vi "Autonomous Independent.vi"() -> ()   [LabVIEW 2015]
doc: "This VI is called when autonomous begins, and will automatically be terminated when autonomous ends. You can carry out timed or sensor driven robot movement independently without needing to return to the caller."
uses:
  <vilib>/Rock Robotics/WPI/Utilities/WPI_GetSetVariantRefNum.vi
  <vilib>/Rock Robotics/Network Tables/NT Read String.vi
  <vilib>/Rock Robotics/Network Tables/NT Write Numeric Array.vi
  <vilib>/Rock Robotics/Network Tables/NT Write Number.vi
  <vilib>/addons/control/pid/pid.llb/PID (DBL).vi
  Robot Global Data.vi
  <vilib>/Rock Robotics/Network Tables/NT Read Number.vi
  <vilib>/addons/control/pid/NI_PID_pid.lvlib
  navX Library v2/navX Library v2.lvlib
panel:
  in  "Aiming Gains":T1={"proportional gain (Kc)"=1.0, "integral time (Ti, min)"=0.01, "derivative time (Td, min)"=0.0} {"derivative time (Td, min)" format="%.3f"; "integral time (Ti, min)" format="%.3f"; "proportional gain (Kc)" format="%.3f"}
  out "Yaw":dbl(graph)
  in  "Target Angle":dbl=30.0
  out "E1 Rate":dbl
  out "E2 Rate":dbl
  out "Yaw Display":dbl
  in  "Single Turn Gains":T1={"proportional gain (Kc)"=0.12, "integral time (Ti, min)"=0.0, "derivative time (Td, min)"=0.0} {"derivative time (Td, min)" format="%.3f"; "integral time (Ti, min)" format="%.3f"; "proportional gain (Kc)" format="%.3f"}
  in  "Yaw":T1={"proportional gain (Kc)"=0.2, "integral time (Ti, min)"=0.0, "derivative time (Td, min)"=0.0} {"derivative time (Td, min)" format="%.3f"; "integral time (Ti, min)" format="%.3f"; "proportional gain (Kc)" format="%.3f"}
  out "Right Motor Speed":dbl(graph)
  out "Left Motor Speed":dbl(graph)
  out "Right Motor":dbl(graph)
  out "Left Motor":dbl(graph)
  in  "Distance":dbl=120.0
  in  "Speed Gains":T1={"proportional gain (Kc)"=0.65, "integral time (Ti, min)"=0.001, "derivative time (Td, min)"=0.001} {"derivative time (Td, min)" format="%.3f"; "integral time (Ti, min)" format="%.3f"; "proportional gain (Kc)" format="%.3f"}
  out "E2 Dist":dbl
  out "E1 Dist":dbl
  # "Be sure to right-click and choose Data Operations>>Make Current Value default if you want to save the array values with the VI"
  # "Encoder Distance Traveled"
  # "Speed we are assigning the motors and Encoder Rate"
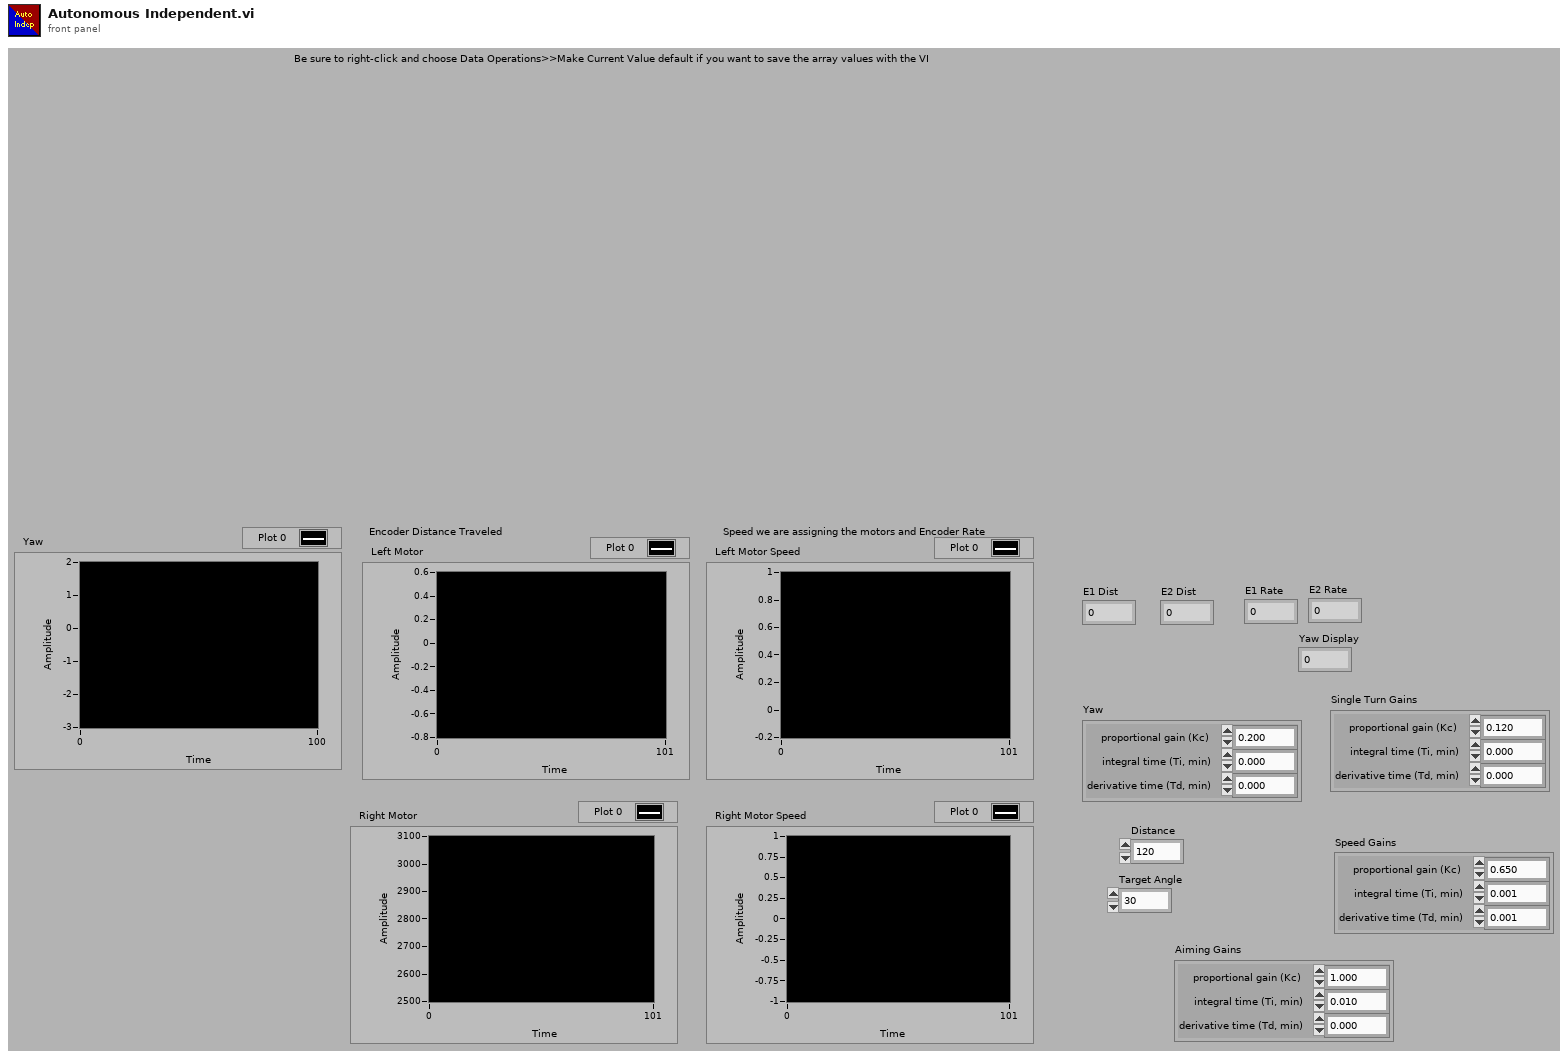
[diagram p1: front panel]
types:
  T1 = cluster{"proportional gain (Kc)":dbl, "integral time (Ti, min)":dbl, "derivative time (Td, min)":dbl}
  T2 = typedef "WPI_JoystickDevRef.ctl" = cluster{"Device":T3}
  T3 = typedef "WPI_JoystickDeviceEnum.ctl" = enum16{"USB 0", "USB 1", "USB 2", "USB 3", "USB 4", "USB 5"}
  T4 = typedef "navX Library v2.lvlib/Z900_navX_DeviceTypeDef.ctl" = cluster{"Interface":cluster{"Protocol":T5, "Update Rate (4Hz-60Hz)":u8, "navX Open TypeDef":variant}, "Notify Packet":refnum<notifier>, "Loop VI Refnum":refnum<vi>, "Ready to Close Occurrence Refnum":refnum<k4>}
  T5 = typedef "navX Library v2.lvlib/Z900_navX_ProtocolTypeDef.ctl" = enum16{"SERIAL", "I2C", "SPI"}
  T6 = typedef "WPI_EncoderDevRef.ctl" = cluster{"DevStatus":errorcluster, "EncoderIndex":T7, "CounterIndex":T8, "DistancePerCount":dbl, "Decoding Type":T9}
  T7 = typedef "FPGA_EncoderIdx.ctl" = enum8{"Enc 0", "Enc 1", "Enc 2", "Enc 3", "Enc 4", "Enc 5", "Enc 6", "Enc 7", "Invalid"}
  T8 = typedef "FPGA_CounterCtrSystemIndex.ctl" = enum8{"Ctr 0", "Ctr 1", "Ctr 2", "Ctr 3", "Ctr 4", "Ctr 5", "Ctr 6", "Ctr 7", "Invalid"}
  T9 = typedef "WPI_EncoderType.ctl" = enum16{"1x", "2x", "4x"}
  T10 = cluster{"Yaw":dbl, "Roll":dbl, "Pitch":dbl, "Heading":dbl, "Fused Heading":dbl}
  T11 = typedef "WPI_RobotDriveDevRef.ctl" = cluster{"DevStatus":errorcluster, "Motors[]":T12[], "Square Inputs":bool, "Max Output":dbl}
  T12 = typedef "WPI_MotorControlDeviceRef.ctl" = cluster{"DeviceStatus":errorcluster, "Type":T13, "PWM":cluster{"PWM Channel":T14, "DeadBand":T15}, "CAN":cluster{"Device Number":u8, "Control Mode":T16, "Semaphore":T17, "Max Vout":dbl, "TalonSRX Control Mode":T18}, "Invert":bool}
  T13 = typedef "WPI_MotorControlType.ctl" = enum16{"PWM", "CAN", "CANTalonSRX"}
  T14 = typedef "FPGA_DIOPWMChannel.ctl" = enum8{"PWM 0", "PWM 1", "PWM 2", "PWM 3", "PWM 4", "PWM 5", "PWM 6", "PWM 7", "PWM 8", "PWM 9", "PWM MXP 0", "PWM MXP 1", "PWM MXP 2", "PWM MXP 3", "PWM MXP 4", "PWM MXP 5", "PWM MXP 6", "PWM MXP 7", "PWM MXP 8", "PWM MXP 9", "Invalid"}
  T15 = typedef "WPI_PWMDeadband.ctl" = cluster{"Name":string, "maxPositivePwm":i32, "minPositivePwm":i32, "centerPwm":i32, "maxNegativePwm":i32, "minNegativePwm":i32, "angularRange":u16}
  T16 = typedef "WPI_CANJaguar_ControlMode.ctl" = enum8{"Percent VBus", "Current", "Speed", "Position", "Voltage"}
  T17 = typedef "Semaphore RefNum" = refnum<k1>
  T18 = typedef "WPI_CANTalonSRX_APIControlMode.ctl" = enum8{"Percent VBus", "Speed", "Position", "Slave", "Unchanged / Invalid", "Voltage Compensation", "Current", "Motion Profile"}
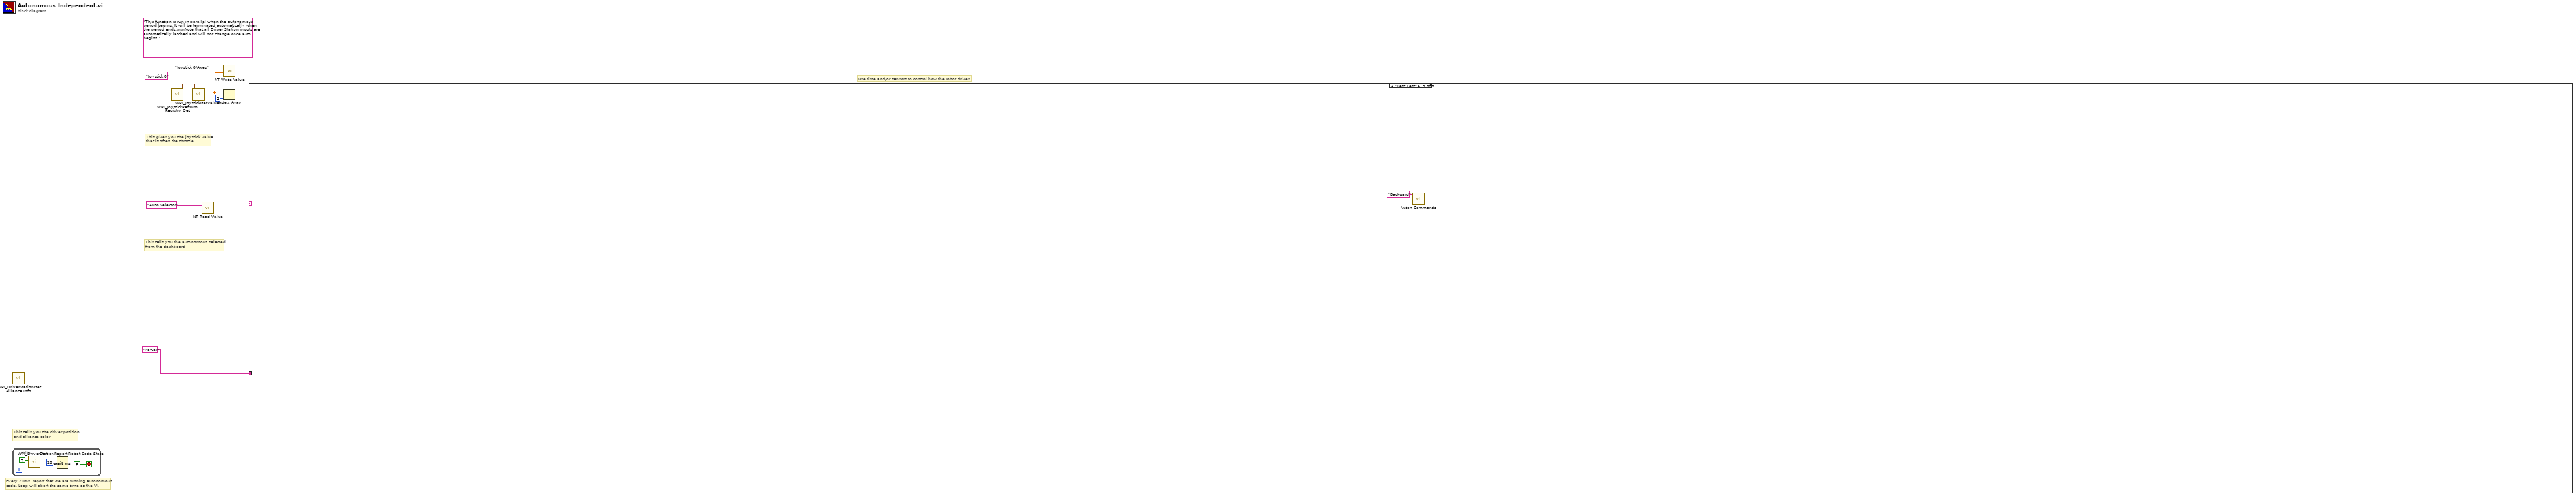
[diagram p0: block diagram]
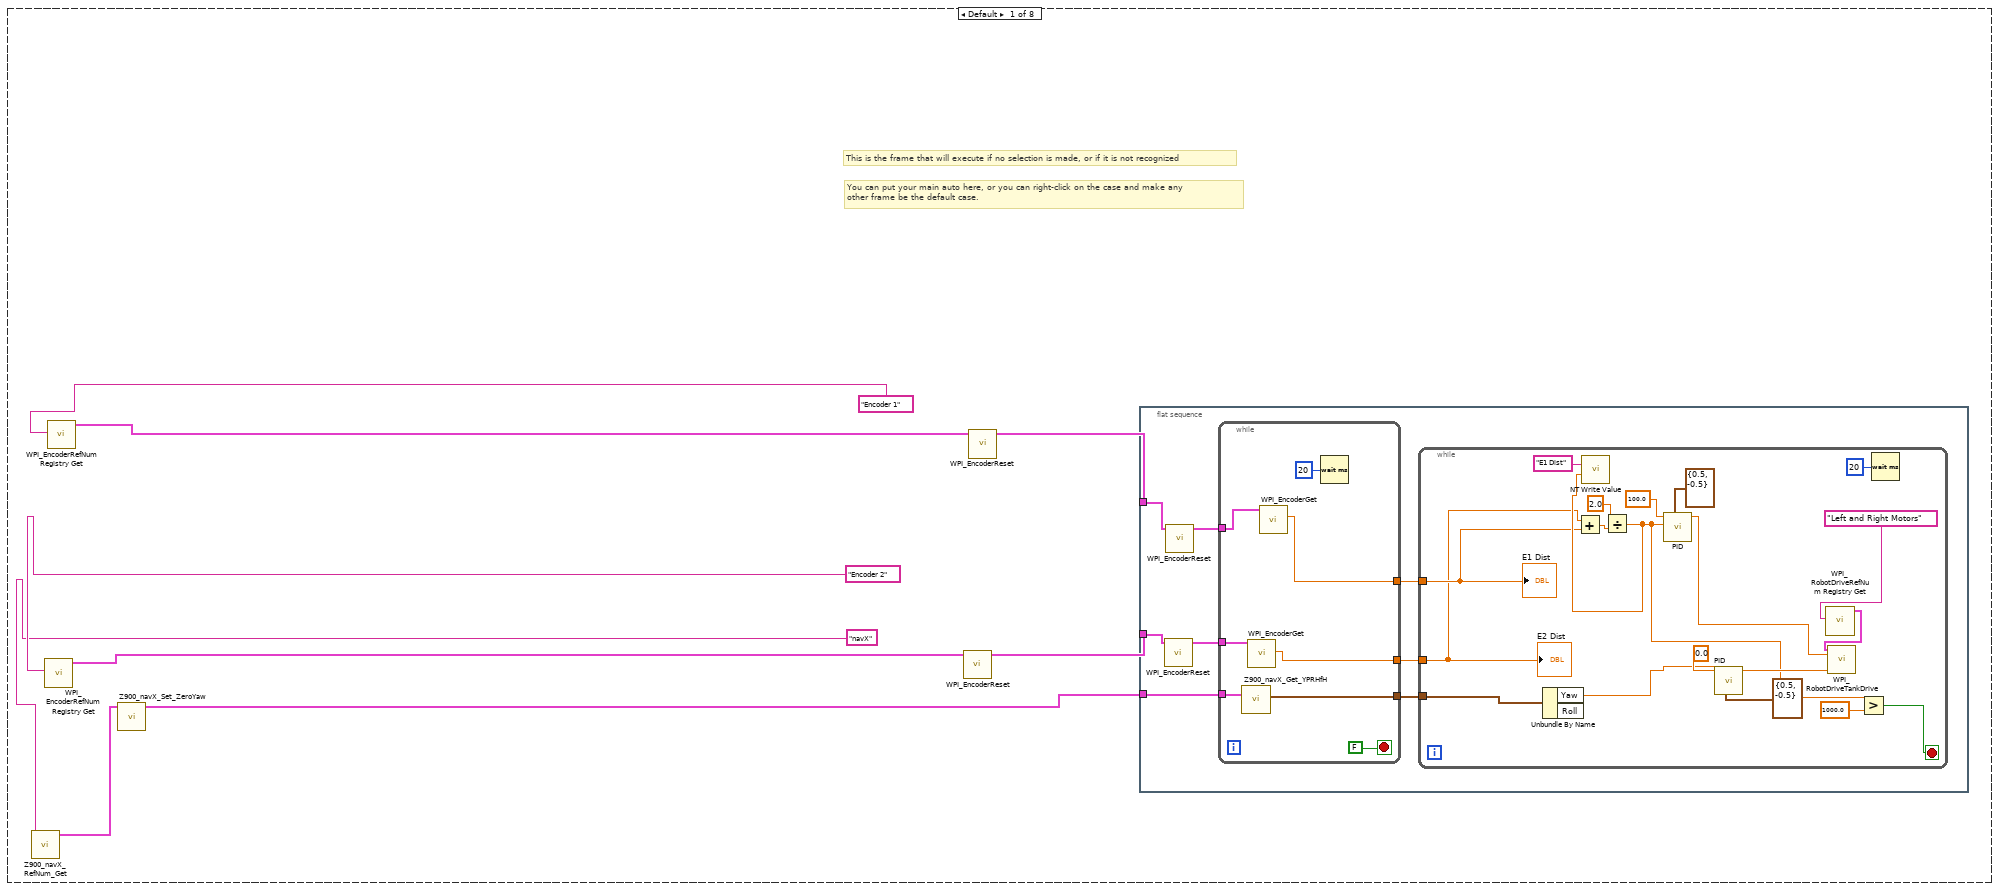
[diagram p2: hidden frame]
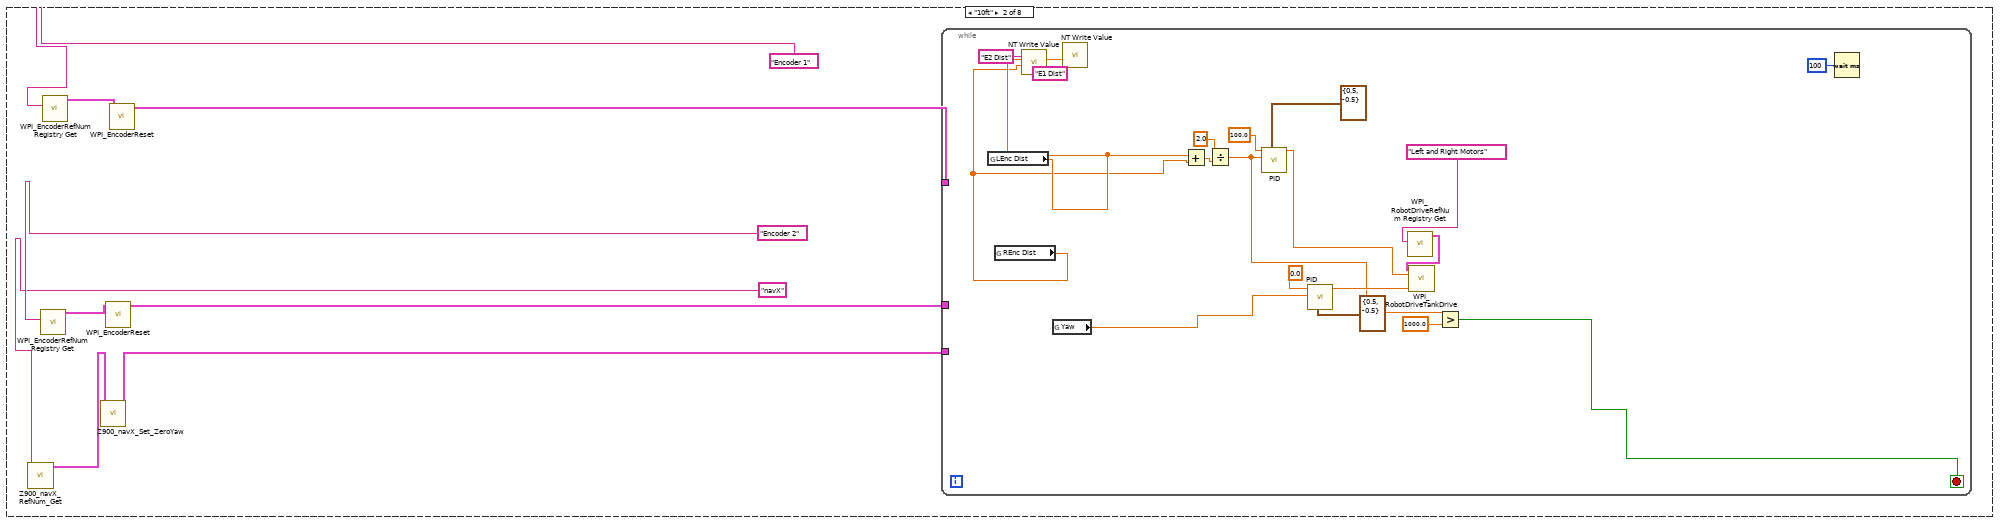
[diagram p3: hidden frame]
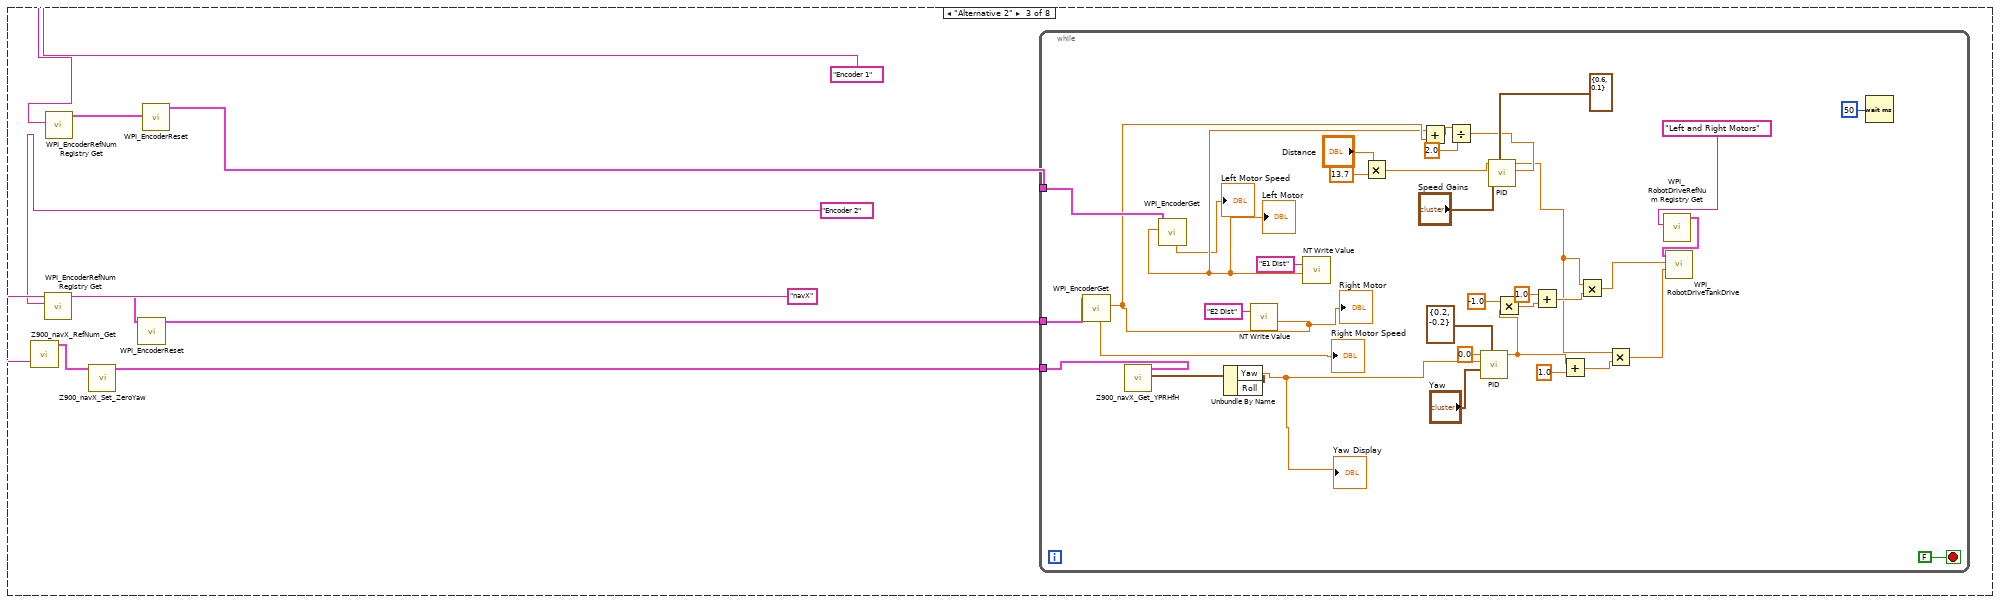
[diagram p4: hidden frame]
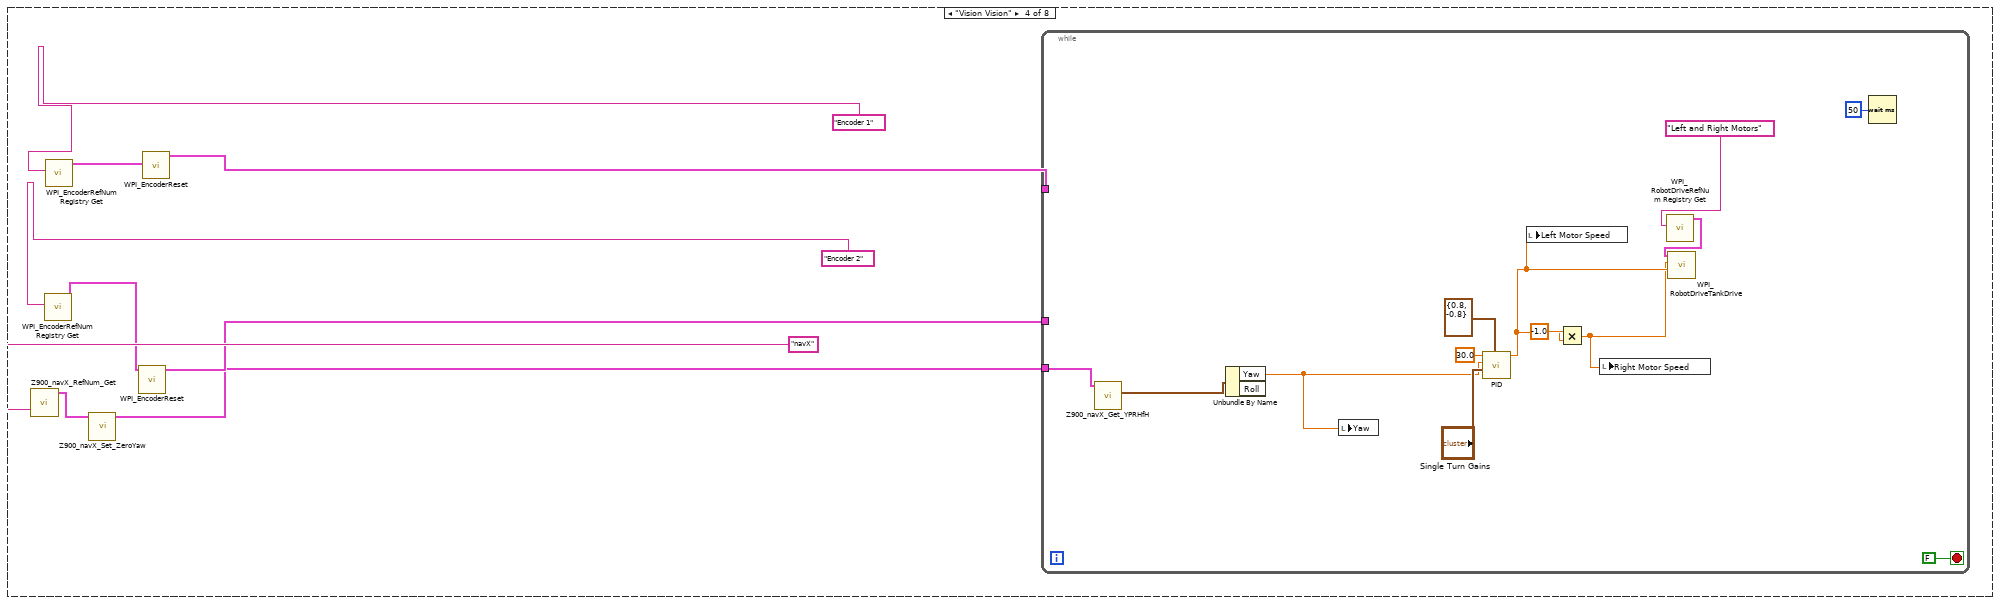
[diagram p5: hidden frame]
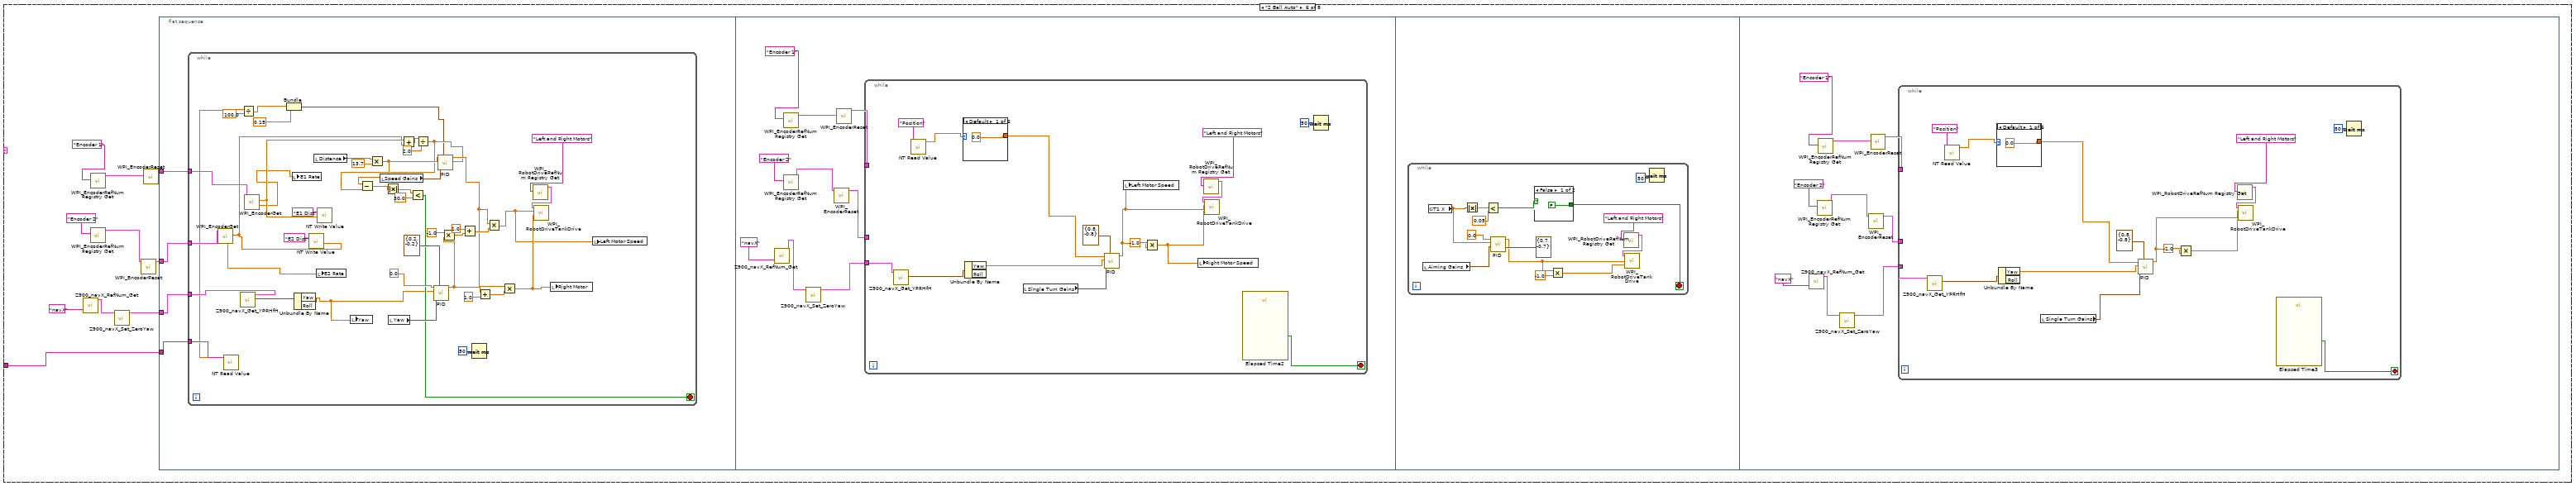
[diagram p6: hidden frame]
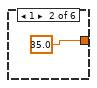
[diagram p7: hidden frame]
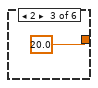
[diagram p8: hidden frame]
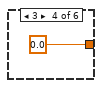
[diagram p9: hidden frame]
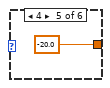
[diagram p10: hidden frame]
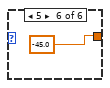
[diagram p11: hidden frame]
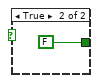
[diagram p12: hidden frame]
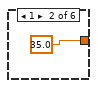
[diagram p13: hidden frame]
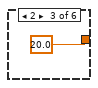
[diagram p14: hidden frame]
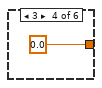
[diagram p15: hidden frame]
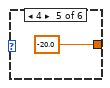
[diagram p16: hidden frame]
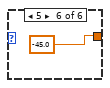
[diagram p17: hidden frame]
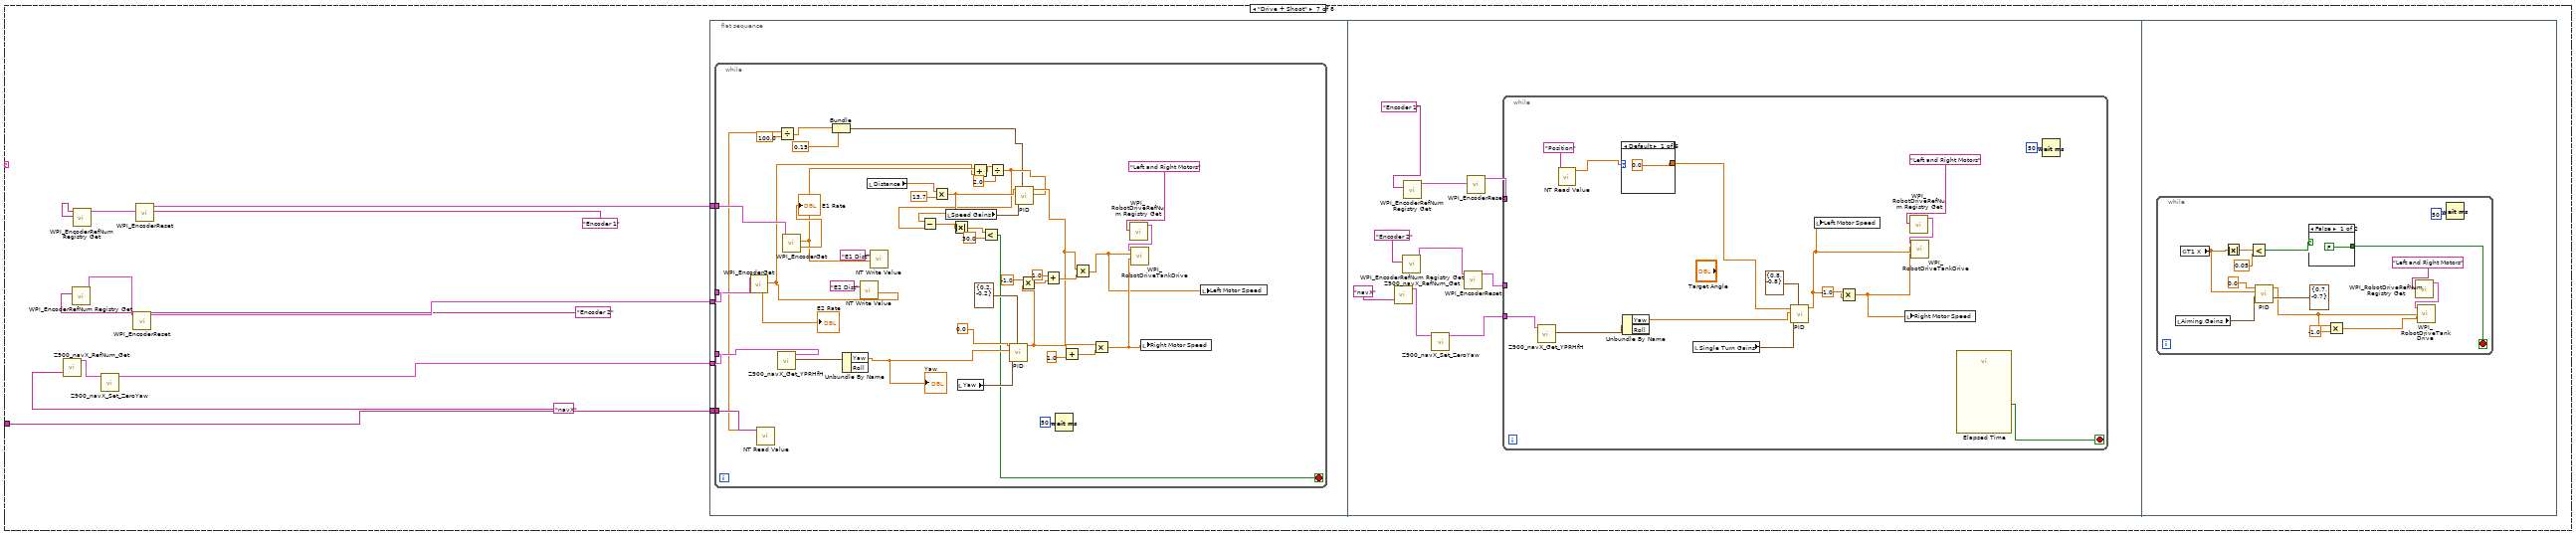
[diagram p18: hidden frame]
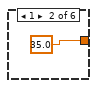
[diagram p19: hidden frame]
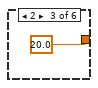
[diagram p20: hidden frame]
diagram:
  (unwired) "This function is run in parallel when the autonomous period begins. It will be terminated automatically when the period ends.\n\nNote that all Driver Station inputs are automatically latched and will not change once auto begins."
  # "This tells you the autonomous selected\nfrom the dashboard"
  # "Every 20ms, report that we are running autonomous\ncode. Loop will abort the same time as the VI."
  # "This gives you the joystick value\nthat is often the throttle"
  # "Use time and/or sensors to control how the robot drives."
  # "This tells you the driver position\nand alliance color"
  n1 = while {
    stop <- FALSE stop-if-true
    n2 = call <vilib>:"WPI_DriverStationReport Robot Code State.vi"("Autonomous"=TRUE) -> ()  [unwired: 10 in, 1 out]
    n3 = Wait (ms)(milliseconds to wait=u32 20) -> ()  [unwired: 1 out]
  }
  n4 = call <vilib>:"WPI_DriverStationGet Alliance Info.vi"() -> ()  [unwired: 12 out]
  n5 = call <vilib>:"WPI_JoystickRefNum Registry Get.vi"("refnum name"="Joystick 0") -> ("JoystickDevRef"=w7:T2)  [unwired: 1 in, 9 out]
  n6 = call <vilib>:"WPI_JoystickGetValues.vi"("JoystickDevRef"=w7) -> ("Axes"=w3:dbl[])  [unwired: 6 in, 4 out]
  n7 = call-poly <vilib>:"NT Read Value.vi"("Name"="Auto Selector") -> ("String"=w4:string)  [unwired: 9 in, 1 out]
  n8 = call-poly <vilib>:"NT Write Value.vi"("Numeric Array"=w3, "Name"="Joystick 0/Axes") -> ()  [unwired: 9 in, 1 out]
  n9 = Index Array(array=w3, index=2) -> ()  [unwired: 1 out]
  n10 = case shown="\"Test Test\"" w4 {
    tunnel: "Power" ("Name") -> [_ _ _ _ _ w152 w286 _]
    frame Default {
      # "You can put your main auto here, or you can right-click on the case and make any\nother frame be the default case."
      # "This is the frame that will execute if no selection is made, or if it is not recognized"
      n11 = call "Z900_navX_RefNum_Get.vi"("refnum name"="navX") -> ("navX Device"=w14:T4)  [unwired: 9 in, 1 out]
      n12 = call <vilib>:"WPI_EncoderRefNum Registry Get.vi"("refnum name"="Encoder 2") -> ("EncoderDevRef"=w16:T6)  [unwired: 9 in, 1 out]
      n13 = call <vilib>:"WPI_EncoderRefNum Registry Get.vi"("refnum name"="Encoder 1") -> ("EncoderDevRef"=w18:T6)  [unwired: 9 in, 1 out]
      n14 = call "Z900_navX_Set_ZeroYaw.vi"("navX Device"=w14) -> ("navX Device"=w13:T4)  [unwired: 9 in, 1 out]
      n15 = call <vilib>:"WPI_EncoderReset.vi"("EncoderDevRef"=w16) -> ("EncoderDevRef"=w15:T6)  [unwired: 9 in, 1 out]
      n16 = call <vilib>:"WPI_EncoderReset.vi"("EncoderDevRef"=w18) -> ("EncoderDevRef"=w17:T6)  [unwired: 9 in, 1 out]
      n17 = flat-sequence {
        tunnel: w17 -> [w28]
        tunnel: w15 -> [w27]
        tunnel: w13 -> [w26]
        frame #0 {
          n18 = call <vilib>:"WPI_EncoderReset.vi"("EncoderDevRef"=w27) -> ("EncoderDevRef"=w25:T6)  [unwired: 9 in, 1 out]
          n19 = call <vilib>:"WPI_EncoderReset.vi"("EncoderDevRef"=w28) -> ("EncoderDevRef"=w24:T6)  [unwired: 9 in, 1 out]
          n20 = while {
            tunnel: w26 -> [w33]
            tunnel: w25 -> [w34]
            tunnel: w24 -> [w35]
            tunnel: [w32] -> w23
            tunnel: [w31] -> w22
            tunnel: [w30] -> w21
            stop <- FALSE stop-if-true
            n21 = call "Z900_navX_Get_YPRHfH.vi"("navX Device"=w33) -> ("YRPHfH"=w32:T10)  [unwired: 7 in, 3 out]
            n22 = call <vilib>:"WPI_EncoderGet.vi"("EncoderDevRef"=w34) -> ("Distance"=w31:dbl)  [unwired: 5 in, 5 out]
            n23 = call <vilib>:"WPI_EncoderGet.vi"("EncoderDevRef"=w35) -> ("Distance"=w30:dbl)  [unwired: 5 in, 5 out]
            n24 = Wait (ms)(milliseconds to wait=u32 20) -> ()  [unwired: 1 out]
          }
          n25 = while {
            tunnel: w23 -> [w40]
            tunnel: w22 -> [w38]
            tunnel: w21 -> [w39]
            stop <- w44 stop-if-true
            n26 = Unbundle By Name(w40) -> ("Yaw"=w41:dbl)  [unwired: 1 out]
            n27 = Add(x=w38, y=w39) -> (x+y=w55:dbl)
            n28 = Divide(x=2.0, y=w55) -> (x/y=w43:dbl)
            n29 = call-poly <vilib>:"NT Write Value.vi"("Numeric"=w43, "Name"="E1 Dist") -> ()  [unwired: 9 in, 1 out]
            n30 = call-poly <vilib>:"PID.vi"("output range"=cluster{"output high":dbl, "output low":dbl} {"output high"=0.5, "output low"=-0.5}, "process variable"=w43, "setpoint"=100.0) -> ("output"=w48:dbl)  [unwired: 7 in, 1 out]
            n31 = call-poly <vilib>:"PID.vi"("output range"=cluster{"output high":dbl, "output low":dbl} {"output high"=0.5, "output low"=-0.5}, "process variable"=w41, "setpoint"=0.0) -> ("output"=w47:dbl)  [unwired: 7 in, 1 out]
            n32 = call <vilib>:"WPI_RobotDriveRefNum Registry Get.vi"("refnum name"="Left and Right Motors") -> ("RobotDriveDevRef"=w50:T11)  [unwired: 9 in, 1 out]
            n33 = call <vilib>:"WPI_RobotDriveTankDrive.vi"("Right axis value"=w47, "Left axis value"=w48, "RobotDriveDevRef"=w50) -> ()  [unwired: 6 in, 3 out]
            n34 = Greater?(x=w43, y=1000.0) -> (0:w44:bool)
            n35 = Wait (ms)(milliseconds to wait=u32 20) -> ()  [unwired: 1 out]
            "E2 Dist" <- w38
            "E1 Dist" <- w39
          }
        }
      }
    }
    frame "10ft" {
      n36 = call "Z900_navX_RefNum_Get.vi"("refnum name"="navX") -> ("navX Device"=w58:T4)  [unwired: 9 in, 1 out]
      n37 = call <vilib>:"WPI_EncoderRefNum Registry Get.vi"("refnum name"="Encoder 2") -> ("EncoderDevRef"=w60:T6)  [unwired: 9 in, 1 out]
      n38 = call <vilib>:"WPI_EncoderRefNum Registry Get.vi"("refnum name"="Encoder 1") -> ("EncoderDevRef"=w62:T6)  [unwired: 9 in, 1 out]
      n39 = call "Z900_navX_Set_ZeroYaw.vi"("navX Device"=w58) -> ("navX Device"=w57:T4)  [unwired: 9 in, 1 out]
      n40 = call <vilib>:"WPI_EncoderReset.vi"("EncoderDevRef"=w60) -> ("EncoderDevRef"=w59:T6)  [unwired: 9 in, 1 out]
      n41 = call <vilib>:"WPI_EncoderReset.vi"("EncoderDevRef"=w62) -> ("EncoderDevRef"=w61:T6)  [unwired: 9 in, 1 out]
      n42 = while {
        tunnel: w61 -> [_]
        tunnel: w59 -> [_]
        tunnel: w57 -> [_]
        stop <- w65 stop-if-true
        n43 = global read "Robot Global Data.vi" "LEnc Dist"() -> (w68:dbl)
        n44 = global read "Robot Global Data.vi" "REnc Dist"() -> (w67:dbl)
        n45 = call-poly <vilib>:"NT Write Value.vi"("Numeric"=w67, "Name"="E2 Dist") -> ()  [unwired: 9 in, 1 out]
        n46 = global read "Robot Global Data.vi" "Yaw"() -> (w66:dbl)
        n47 = call-poly <vilib>:"NT Write Value.vi"("Numeric"=w68, "Name"="E1 Dist") -> ()  [unwired: 9 in, 1 out]
        n48 = Add(x=w68, y=w67) -> (x+y=w82:dbl)
        n49 = Divide(x=2.0, y=w82) -> (x/y=w72:dbl)
        n50 = call-poly <vilib>:"PID.vi"("output range"=cluster{"output high":dbl, "output low":dbl} {"output high"=0.5, "output low"=-0.5}, "process variable"=w72, "setpoint"=100.0) -> ("output"=w76:dbl)  [unwired: 7 in, 1 out]
        n51 = call-poly <vilib>:"PID.vi"("output range"=cluster{"output high":dbl, "output low":dbl} {"output high"=0.5, "output low"=-0.5}, "process variable"=w66, "setpoint"=0.0) -> ("output"=w75:dbl)  [unwired: 7 in, 1 out]
        n52 = call <vilib>:"WPI_RobotDriveRefNum Registry Get.vi"("refnum name"="Left and Right Motors") -> ("RobotDriveDevRef"=w78:T11)  [unwired: 9 in, 1 out]
        n53 = call <vilib>:"WPI_RobotDriveTankDrive.vi"("Right axis value"=w75, "Left axis value"=w76, "RobotDriveDevRef"=w78) -> ()  [unwired: 6 in, 3 out]
        n54 = Greater?(x=w72, y=1000.0) -> (0:w65:bool)
        n55 = Wait (ms)(milliseconds to wait=u32 100) -> ()  [unwired: 1 out]
      }
    }
    frame "Alternative 2" {
      n56 = call "Z900_navX_RefNum_Get.vi"("refnum name"="navX") -> ("navX Device"=w85:T4)  [unwired: 9 in, 1 out]
      n57 = call <vilib>:"WPI_EncoderRefNum Registry Get.vi"("refnum name"="Encoder 2") -> ("EncoderDevRef"=w87:T6)  [unwired: 9 in, 1 out]
      n58 = call <vilib>:"WPI_EncoderRefNum Registry Get.vi"("refnum name"="Encoder 1") -> ("EncoderDevRef"=w89:T6)  [unwired: 9 in, 1 out]
      n59 = call "Z900_navX_Set_ZeroYaw.vi"("navX Device"=w85) -> ("navX Device"=w84:T4)  [unwired: 9 in, 1 out]
      n60 = call <vilib>:"WPI_EncoderReset.vi"("EncoderDevRef"=w87) -> ("EncoderDevRef"=w86:T6)  [unwired: 9 in, 1 out]
      n61 = call <vilib>:"WPI_EncoderReset.vi"("EncoderDevRef"=w89) -> ("EncoderDevRef"=w88:T6)  [unwired: 9 in, 1 out]
      n62 = while {
        tunnel: w88 -> [w121]
        tunnel: w86 -> [w120]
        tunnel: w84 -> [w119]
        stop <- FALSE stop-if-true
        n63 = call <vilib>:"WPI_EncoderGet.vi"("EncoderDevRef"=w120) -> ("Distance"=w110:dbl, "Rate"=→"Right Motor Speed":dbl)  [unwired: 5 in, 4 out]
        "Right Motor" <- w110
        n64 = call "Z900_navX_Get_YPRHfH.vi"("navX Device"=w119) -> ("YRPHfH"=w122:T10)  [unwired: 7 in, 3 out]
        n65 = call <vilib>:"WPI_EncoderGet.vi"("EncoderDevRef"=w121) -> ("Distance"=w109:dbl, "Rate"=→"Left Motor Speed":dbl)  [unwired: 5 in, 4 out]
        "Left Motor" <- w109
        n66 = Unbundle By Name(w122) -> ("Yaw"=w95:dbl)  [unwired: 1 out]
        "Yaw Display" <- w95
        n67 = call-poly <vilib>:"NT Write Value.vi"("Numeric"=w110, "Name"="E2 Dist") -> ()  [unwired: 9 in, 1 out]
        n68 = call-poly <vilib>:"NT Write Value.vi"("Numeric"=w109, "Name"="E1 Dist") -> ()  [unwired: 9 in, 1 out]
        n69 = Multiply(x="Distance", y=13.7) -> (x*y=w111:dbl)
        n70 = Add(x=w109, y=w110) -> (x+y=w116:dbl)
        n71 = Divide(x=w116, y=2.0) -> (x/y=w114:dbl)
        n72 = call-poly <vilib>:"PID.vi"("output range"=cluster{"output high":dbl, "output low":dbl} {"output high"=0.2, "output low"=-0.2}, "PID gains"="Yaw", "process variable"=w95, "setpoint"=0.0) -> ("output"=w99:dbl)  [unwired: 6 in, 1 out]
        n73 = call-poly <vilib>:"PID.vi"("output range"=cluster{"output high":dbl, "output low":dbl} {"output high"=0.6, "output low"=0.1}, "PID gains"="Speed Gains", "process variable"=w114, "setpoint"=w111) -> ("output"=w96:dbl)  [unwired: 6 in, 1 out]
        n74 = Multiply(x=-1.0, y=w99) -> (x*y=w100:dbl)
        n75 = Add(x=1.0, y=w100) -> (x+y=w101:dbl)
        n76 = Add(x=w99, y=1.0) -> (x+y=w102:dbl)
        n77 = Multiply(x=w96, y=w101) -> (x*y=w93:dbl)
        n78 = Multiply(x=w96, y=w102) -> (x*y=w94:dbl)
        n79 = call <vilib>:"WPI_RobotDriveRefNum Registry Get.vi"("refnum name"="Left and Right Motors") -> ("RobotDriveDevRef"=w124:T11)  [unwired: 9 in, 1 out]
        n80 = call <vilib>:"WPI_RobotDriveTankDrive.vi"("Right axis value"=w94, "Left axis value"=w93, "RobotDriveDevRef"=w124) -> ()  [unwired: 6 in, 3 out]
        n81 = Wait (ms)(milliseconds to wait=u32 50) -> ()  [unwired: 1 out]
      }
    }
    frame "Vision Vision" {
      n82 = call "Z900_navX_RefNum_Get.vi"("refnum name"="navX") -> ("navX Device"=w130:T4)  [unwired: 9 in, 1 out]
      n83 = call <vilib>:"WPI_EncoderRefNum Registry Get.vi"("refnum name"="Encoder 2") -> ("EncoderDevRef"=w132:T6)  [unwired: 9 in, 1 out]
      n84 = call <vilib>:"WPI_EncoderRefNum Registry Get.vi"("refnum name"="Encoder 1") -> ("EncoderDevRef"=w134:T6)  [unwired: 9 in, 1 out]
      n85 = call "Z900_navX_Set_ZeroYaw.vi"("navX Device"=w130) -> ("navX Device"=w129:T4)  [unwired: 9 in, 1 out]
      n86 = call <vilib>:"WPI_EncoderReset.vi"("EncoderDevRef"=w132) -> ("EncoderDevRef"=w131:T6)  [unwired: 9 in, 1 out]
      n87 = call <vilib>:"WPI_EncoderReset.vi"("EncoderDevRef"=w134) -> ("EncoderDevRef"=w133:T6)  [unwired: 9 in, 1 out]
      n88 = while {
        tunnel: w133 -> [_]
        tunnel: w131 -> [_]
        tunnel: w129 -> [w144]
        stop <- FALSE stop-if-true
        n89 = call "Z900_navX_Get_YPRHfH.vi"("navX Device"=w144) -> ("YRPHfH"=w143:T10)  [unwired: 7 in, 3 out]
        n90 = Unbundle By Name(w143) -> ("Yaw"=w138:dbl)  [unwired: 1 out]
        n91 = local write "Yaw"(w138) -> ()
        n92 = call-poly <vilib>:"PID.vi"("output range"=cluster{"output high":dbl, "output low":dbl} {"output high"=0.8, "output low"=-0.8}, "PID gains"="Single Turn Gains", "process variable"=w138, "setpoint"=30.0) -> ("output"=w140:dbl)  [unwired: 6 in, 1 out]
        n93 = local write "Left Motor Speed"(w140) -> ()
        n94 = Multiply(x=-1.0, y=w140) -> (x*y=w139:dbl)
        n95 = local write "Right Motor Speed"(w139) -> ()
        n96 = call <vilib>:"WPI_RobotDriveRefNum Registry Get.vi"("refnum name"="Left and Right Motors") -> ("RobotDriveDevRef"=w149:T11)  [unwired: 9 in, 1 out]
        n97 = call <vilib>:"WPI_RobotDriveTankDrive.vi"("Right axis value"=w140, "Left axis value"=w139, "RobotDriveDevRef"=w149) -> ()  [unwired: 6 in, 3 out]
        n98 = Wait (ms)(milliseconds to wait=u32 50) -> ()  [unwired: 1 out]
      }
    }
    frame "Test Test" {
      n99 = call "Auton Commands.vi"("Task"="Backward") -> ()  [unwired: 10 in]
    }
    frame "2 Ball Auto" {
      n100 = call "Z900_navX_RefNum_Get.vi"("refnum name"="navX") -> ("navX Device"=w160:T4)  [unwired: 9 in, 1 out]
      n101 = call <vilib>:"WPI_EncoderRefNum Registry Get.vi"("refnum name"="Encoder 2") -> ("EncoderDevRef"=w158:T6)  [unwired: 9 in, 1 out]
      n102 = call <vilib>:"WPI_EncoderRefNum Registry Get.vi"("refnum name"="Encoder 1") -> ("EncoderDevRef"=w156:T6)  [unwired: 9 in, 1 out]
      n103 = call "Z900_navX_Set_ZeroYaw.vi"("navX Device"=w160) -> ("navX Device"=w161:T4)  [unwired: 9 in, 1 out]
      n104 = call <vilib>:"WPI_EncoderReset.vi"("EncoderDevRef"=w158) -> ("EncoderDevRef"=w159:T6)  [unwired: 9 in, 1 out]
      n105 = call <vilib>:"WPI_EncoderReset.vi"("EncoderDevRef"=w156) -> ("EncoderDevRef"=w157:T6)  [unwired: 9 in, 1 out]
      n106 = flat-sequence {
        tunnel: w161 -> [w165]
        tunnel: w159 -> [w164]
        tunnel: w157 -> [w163]
        tunnel: w152 -> [w162]
        frame #0 {
          n107 = while {
            tunnel: w163 -> [w203]
            tunnel: w164 -> [w202]
            tunnel: w165 -> [w201]
            tunnel: w162 -> [w175]
            stop <- w176 stop-if-true
            n108 = call <vilib>:"WPI_EncoderGet.vi"("EncoderDevRef"=w202) -> ("Distance"=w182:dbl, "Rate"=w167:dbl)  [unwired: 5 in, 4 out]
            n109 = call-poly <vilib>:"NT Read Value.vi"("Name"=w175) -> ("Numeric"=w174:dbl)  [unwired: 9 in, 1 out]
            n110 = call "Z900_navX_Get_YPRHfH.vi"("navX Device"=w201) -> ("YRPHfH"=w204:T10)  [unwired: 7 in, 3 out]
            n111 = Divide(x=w174, y=100.0) -> (x/y=w172:dbl)
            n112 = call <vilib>:"WPI_EncoderGet.vi"("EncoderDevRef"=w203) -> ("Distance"=w183:dbl, "Rate"=w166:dbl)  [unwired: 5 in, 4 out]
            n113 = Bundle(w172, "output low"=0.15) -> (w170:cluster{dbl, "output low":dbl})  [unwired: 1 in]
            n114 = local write "E1 Rate"(w166) -> ()
            n115 = Unbundle By Name(w204) -> ("Yaw"=w168:dbl)  [unwired: 1 out]
            n116 = call-poly <vilib>:"NT Write Value.vi"("Numeric"=w182, "Name"="E2 Dist") -> ()  [unwired: 9 in, 1 out]
            n117 = local read "Distance"() -> (w169:dbl)
            n118 = local write "E2 Rate"(w167) -> ()
            n119 = call-poly <vilib>:"NT Write Value.vi"("Numeric"=w183, "Name"="E1 Dist") -> ()  [unwired: 9 in, 1 out]
            n120 = local write "Yaw"(w168) -> ()
            n121 = Multiply(x=w169, y=13.7) -> (x*y=w181:dbl)
            n122 = local read "Speed Gains"() -> (w185:T1)
            n123 = local read "Yaw"() -> (w188:T1)
            n124 = Add(x=w183, y=w182) -> (x+y=w200:dbl)
            n125 = Divide(x=w200, y=2.0) -> (x/y=w180:dbl)
            n126 = Subtract(x=w181, y=w180) -> (x-y=w179:dbl)
            n127 = Absolute Value(x=w179) -> (abs(x)=w178:dbl)
            n128 = Less?(x=w178, y=30.0) -> (x < y?=w176:bool)
            n129 = call-poly <vilib>:"PID.vi"("output range"=cluster{"output high":dbl, "output low":dbl} {"output high"=0.2, "output low"=-0.2}, "PID gains"=w188, "process variable"=w168, "setpoint"=0.0) -> ("output"=w193:dbl)  [unwired: 6 in, 1 out]
            n130 = call-poly <vilib>:"PID.vi"("output range"=w170, "PID gains"=w185, "process variable"=w180, "setpoint"=w181) -> ("output"=w190:dbl)  [unwired: 6 in, 1 out]
            n131 = Multiply(x=-1.0, y=w193) -> (x*y=w194:dbl)
            n132 = Add(x=1.0, y=w194) -> (x+y=w195:dbl)
            n133 = Wait (ms)(milliseconds to wait=u32 50) -> ()  [unwired: 1 out]
            n134 = Add(x=w193, y=1.0) -> (x+y=w196:dbl)
            n135 = Multiply(x=w190, y=w195) -> (x*y=w186:dbl)
            n136 = Multiply(x=w190, y=w196) -> (x*y=w187:dbl)
            n137 = call <vilib>:"WPI_RobotDriveRefNum Registry Get.vi"("refnum name"="Left and Right Motors") -> ("RobotDriveDevRef"=w206:T11)  [unwired: 9 in, 1 out]
            n138 = call <vilib>:"WPI_RobotDriveTankDrive.vi"("Right axis value"=w187, "Left axis value"=w186, "RobotDriveDevRef"=w206) -> ()  [unwired: 6 in, 3 out]
            n139 = local write "Right Motor"(w187) -> ()
            n140 = local write "Left Motor Speed"(w186) -> ()
          }
        }
        frame #1 {
          n141 = call "Z900_navX_RefNum_Get.vi"("refnum name"="navX") -> ("navX Device"=w211:T4)  [unwired: 9 in, 1 out]
          n142 = call <vilib>:"WPI_EncoderRefNum Registry Get.vi"("refnum name"="Encoder 2") -> ("EncoderDevRef"=w213:T6)  [unwired: 9 in, 1 out]
          n143 = call <vilib>:"WPI_EncoderRefNum Registry Get.vi"("refnum name"="Encoder 1") -> ("EncoderDevRef"=w215:T6)  [unwired: 9 in, 1 out]
          n144 = call "Z900_navX_Set_ZeroYaw.vi"("navX Device"=w211) -> ("navX Device"=w210:T4)  [unwired: 9 in, 1 out]
          n145 = call <vilib>:"WPI_EncoderReset.vi"("EncoderDevRef"=w213) -> ("EncoderDevRef"=w212:T6)  [unwired: 9 in, 1 out]
          n146 = call <vilib>:"WPI_EncoderReset.vi"("EncoderDevRef"=w215) -> ("EncoderDevRef"=w214:T6)  [unwired: 9 in, 1 out]
          n147 = while {
            tunnel: w214 -> [_]
            tunnel: w212 -> [_]
            tunnel: w210 -> [w229]
            stop <- w222 stop-if-true
            n148 = call "Z900_navX_Get_YPRHfH.vi"("navX Device"=w229) -> ("YRPHfH"=w228:T10)  [unwired: 7 in, 3 out]
            n149 = call-poly <vilib>:"NT Read Value.vi"("Name"="Position") -> ("Numeric"=w219:dbl)  [unwired: 9 in, 1 out]
            n150 = case shown="Default" w219 {
              tunnel: [0.0 35.0 20.0 0.0 -20.0 -45.0] -> w220
              frame Default {
              }
              frame 1 {
              }
              frame 2 {
              }
              frame 3 {
              }
              frame 4 {
              }
              frame 5 {
              }
            }
            n151 = Unbundle By Name(w228) -> ("Yaw"=w226:dbl)  [unwired: 1 out]
            n152 = local read "Single Turn Gains"() -> (w225:T1)
            n153 = call-poly <vilib>:"PID.vi"("output range"=cluster{"output high":dbl, "output low":dbl} {"output high"=0.8, "output low"=-0.8}, "PID gains"=w225, "process variable"=w226, "setpoint"=w220) -> ("output"=w224:dbl)  [unwired: 6 in, 1 out]
            n154 = local write "Left Motor Speed"(w224) -> ()
            n155 = Multiply(x=-1.0, y=w224) -> (x*y=w223:dbl)
            n156 = local write "Right Motor Speed"(w223) -> ()
            n157 = call <vilib>:"WPI_RobotDriveRefNum Registry Get.vi"("refnum name"="Left and Right Motors") -> ("RobotDriveDevRef"=w232:T11)  [unwired: 9 in, 1 out]
            n158 = call <vilib>:"WPI_RobotDriveTankDrive.vi"("Right axis value"=w224, "Left axis value"=w223, "RobotDriveDevRef"=w232) -> ()  [unwired: 6 in, 3 out]
            n159 = call "Elapsed Time2"() -> ("Time has Elapsed"=w222:bool)  [unwired: 12 in, 7 out]
            n160 = Wait (ms)(milliseconds to wait=u32 50) -> ()  [unwired: 1 out]
          }
        }
        frame #2 {
          n161 = while {
            stop <- w250 stop-if-true
            n162 = local read "Aiming Gains"() -> (w240:T1)
            n163 = global read "Robot Global Data.vi" "T1 X"() -> (w248:dbl)
            n164 = Absolute Value(x=w248) -> (abs(x)=w253:dbl)
            n165 = Less?(x=w253, y=0.05) -> (x < y?=w251:bool)
            n166 = call-poly <vilib>:"PID.vi"("output range"=cluster{"output high":dbl, "output low":dbl} {"output high"=0.7, "output low"=-0.7}, "PID gains"=w240, "process variable"=w248, "setpoint"=0.0) -> ("output"=w242:dbl)  [unwired: 6 in, 1 out]
            n167 = case shown="False" w251 {
              tunnel: [FALSE FALSE] -> w250
              frame False {
              }
              frame True {
              }
            }
            n168 = Multiply(x=w242, y=-1.0) -> (x*y=w241:dbl)
            n169 = call <vilib>:"WPI_RobotDriveRefNum Registry Get.vi"("refnum name"="Left and Right Motors") -> ("RobotDriveDevRef"=w244:T11)  [unwired: 9 in, 1 out]
            n170 = call <vilib>:"WPI_RobotDriveTankDrive.vi"("Right axis value"=w241, "Left axis value"=w242, "RobotDriveDevRef"=w244) -> ()  [unwired: 6 in, 3 out]
            n171 = Wait (ms)(milliseconds to wait=u32 50) -> ()  [unwired: 1 out]
          }
        }
        frame #3 {
          n172 = call "Z900_navX_RefNum_Get.vi"("refnum name"="navX") -> ("navX Device"=w257:T4)  [unwired: 9 in, 1 out]
          n173 = call <vilib>:"WPI_EncoderRefNum Registry Get.vi"("refnum name"="Encoder 2") -> ("EncoderDevRef"=w259:T6)  [unwired: 9 in, 1 out]
          n174 = call <vilib>:"WPI_EncoderRefNum Registry Get.vi"("refnum name"="Encoder 1") -> ("EncoderDevRef"=w261:T6)  [unwired: 9 in, 1 out]
          n175 = call "Z900_navX_Set_ZeroYaw.vi"("navX Device"=w257) -> ("navX Device"=w256:T4)  [unwired: 9 in, 1 out]
          n176 = call <vilib>:"WPI_EncoderReset.vi"("EncoderDevRef"=w259) -> ("EncoderDevRef"=w258:T6)  [unwired: 9 in, 1 out]
          n177 = call <vilib>:"WPI_EncoderReset.vi"("EncoderDevRef"=w261) -> ("EncoderDevRef"=w260:T6)  [unwired: 9 in, 1 out]
          n178 = while {
            tunnel: w260 -> [_]
            tunnel: w258 -> [_]
            tunnel: w256 -> [w275]
            stop <- w269 stop-if-true
            n179 = call "Z900_navX_Get_YPRHfH.vi"("navX Device"=w275) -> ("YRPHfH"=w274:T10)  [unwired: 7 in, 3 out]
            n180 = call-poly <vilib>:"NT Read Value.vi"("Name"="Position") -> ("Numeric"=w266:dbl)  [unwired: 9 in, 1 out]
            n181 = case shown="Default" w266 {
              tunnel: [0.0 35.0 20.0 0.0 -20.0 -45.0] -> w267
              frame Default {
              }
              frame 1 {
              }
              frame 2 {
              }
              frame 3 {
              }
              frame 4 {
              }
              frame 5 {
              }
            }
            n182 = Unbundle By Name(w274) -> ("Yaw"=w272:dbl)  [unwired: 1 out]
            n183 = local read "Single Turn Gains"() -> (w265:T1)
            n184 = call-poly <vilib>:"PID.vi"("output range"=cluster{"output high":dbl, "output low":dbl} {"output high"=0.8, "output low"=-0.8}, "PID gains"=w265, "process variable"=w272, "setpoint"=w267) -> ("output"=w271:dbl)  [unwired: 6 in, 1 out]
            n185 = Multiply(x=-1.0, y=w271) -> (x*y=w270:dbl)
            n186 = call <vilib>:"WPI_RobotDriveRefNum Registry Get.vi"("refnum name"="Left and Right Motors") -> ("RobotDriveDevRef"=w278:T11)  [unwired: 9 in, 1 out]
            n187 = call <vilib>:"WPI_RobotDriveTankDrive.vi"("Right axis value"=w271, "Left axis value"=w270, "RobotDriveDevRef"=w278) -> ()  [unwired: 6 in, 3 out]
            n188 = call "Elapsed Time3"() -> ("Time has Elapsed"=w269:bool)  [unwired: 12 in, 7 out]
            n189 = Wait (ms)(milliseconds to wait=u32 50) -> ()  [unwired: 1 out]
          }
        }
      }
    }
    frame "Drive + Shoot" {
      n190 = call "Z900_navX_RefNum_Get.vi"("refnum name"="navX") -> ("navX Device"=w294:T4)  [unwired: 9 in, 1 out]
      n191 = call <vilib>:"WPI_EncoderRefNum Registry Get.vi"("refnum name"="Encoder 2") -> ("EncoderDevRef"=w292:T6)  [unwired: 9 in, 1 out]
      n192 = call <vilib>:"WPI_EncoderRefNum Registry Get.vi"("refnum name"="Encoder 1") -> ("EncoderDevRef"=w290:T6)  [unwired: 9 in, 1 out]
      n193 = call "Z900_navX_Set_ZeroYaw.vi"("navX Device"=w294) -> ("navX Device"=w295:T4)  [unwired: 9 in, 1 out]
      n194 = call <vilib>:"WPI_EncoderReset.vi"("EncoderDevRef"=w292) -> ("EncoderDevRef"=w293:T6)  [unwired: 9 in, 1 out]
      n195 = call <vilib>:"WPI_EncoderReset.vi"("EncoderDevRef"=w290) -> ("EncoderDevRef"=w291:T6)  [unwired: 9 in, 1 out]
      n196 = flat-sequence {
        tunnel: w295 -> [w299]
        tunnel: w293 -> [w298]
        tunnel: w291 -> [w297]
        tunnel: w286 -> [w296]
        frame #0 {
          n197 = while {
            tunnel: w297 -> [w337]
            tunnel: w298 -> [w336]
            tunnel: w299 -> [w335]
            tunnel: w296 -> [w305]
            stop <- w306 stop-if-true
            n198 = call <vilib>:"WPI_EncoderGet.vi"("EncoderDevRef"=w336) -> ("Distance"=w312:dbl, "Rate"=→"E2 Rate":dbl)  [unwired: 5 in, 4 out]
            n199 = call-poly <vilib>:"NT Read Value.vi"("Name"=w305) -> ("Numeric"=w304:dbl)  [unwired: 9 in, 1 out]
            n200 = call "Z900_navX_Get_YPRHfH.vi"("navX Device"=w335) -> ("YRPHfH"=w338:T10)  [unwired: 7 in, 3 out]
            n201 = Divide(x=w304, y=100.0) -> (x/y=w302:dbl)
            n202 = call <vilib>:"WPI_EncoderGet.vi"("EncoderDevRef"=w337) -> ("Distance"=w313:dbl, "Rate"=→"E1 Rate":dbl)  [unwired: 5 in, 4 out]
            n203 = Bundle(w302, "output low"=0.15) -> (w300:cluster{dbl, "output low":dbl})  [unwired: 1 in]
            n204 = Unbundle By Name(w338) -> ("Yaw"=w314:dbl)  [unwired: 1 out]
            "Yaw" <- w314
            n205 = call-poly <vilib>:"NT Write Value.vi"("Numeric"=w312, "Name"="E2 Dist") -> ()  [unwired: 9 in, 1 out]
            n206 = local read "Distance"() -> (w322:dbl)
            n207 = call-poly <vilib>:"NT Write Value.vi"("Numeric"=w313, "Name"="E1 Dist") -> ()  [unwired: 9 in, 1 out]
            n208 = Multiply(x=w322, y=13.7) -> (x*y=w311:dbl)
            n209 = local read "Speed Gains"() -> (w316:T1)
            n210 = local read "Yaw"() -> (w320:T1)
            n211 = Add(x=w313, y=w312) -> (x+y=w334:dbl)
            n212 = Divide(x=w334, y=2.0) -> (x/y=w310:dbl)
            n213 = Subtract(x=w311, y=w310) -> (x-y=w309:dbl)
            n214 = Absolute Value(x=w309) -> (abs(x)=w308:dbl)
            n215 = Less?(x=w308, y=30.0) -> (x < y?=w306:bool)
            n216 = call-poly <vilib>:"PID.vi"("output range"=cluster{"output high":dbl, "output low":dbl} {"output high"=0.2, "output low"=-0.2}, "PID gains"=w320, "process variable"=w314, "setpoint"=0.0) -> ("output"=w327:dbl)  [unwired: 6 in, 1 out]
            n217 = call-poly <vilib>:"PID.vi"("output range"=w300, "PID gains"=w316, "process variable"=w310, "setpoint"=w311) -> ("output"=w324:dbl)  [unwired: 6 in, 1 out]
            n218 = Multiply(x=-1.0, y=w327) -> (x*y=w328:dbl)
            n219 = Add(x=1.0, y=w328) -> (x+y=w329:dbl)
            n220 = Wait (ms)(milliseconds to wait=u32 50) -> ()  [unwired: 1 out]
            n221 = Add(x=w327, y=1.0) -> (x+y=w330:dbl)
            n222 = Multiply(x=w324, y=w329) -> (x*y=w317:dbl)
            n223 = Multiply(x=w324, y=w330) -> (x*y=w319:dbl)
            n224 = call <vilib>:"WPI_RobotDriveRefNum Registry Get.vi"("refnum name"="Left and Right Motors") -> ("RobotDriveDevRef"=w340:T11)  [unwired: 9 in, 1 out]
            n225 = call <vilib>:"WPI_RobotDriveTankDrive.vi"("Right axis value"=w319, "Left axis value"=w317, "RobotDriveDevRef"=w340) -> ()  [unwired: 6 in, 3 out]
            n226 = local write "Right Motor Speed"(w319) -> ()
            n227 = local write "Left Motor Speed"(w317) -> ()
          }
        }
        frame #1 {
          n228 = call "Z900_navX_RefNum_Get.vi"("refnum name"="navX") -> ("navX Device"=w345:T4)  [unwired: 9 in, 1 out]
          n229 = call <vilib>:"WPI_EncoderRefNum Registry Get.vi"("refnum name"="Encoder 2") -> ("EncoderDevRef"=w347:T6)  [unwired: 9 in, 1 out]
          n230 = call <vilib>:"WPI_EncoderRefNum Registry Get.vi"("refnum name"="Encoder 1") -> ("EncoderDevRef"=w349:T6)  [unwired: 9 in, 1 out]
          n231 = call "Z900_navX_Set_ZeroYaw.vi"("navX Device"=w345) -> ("navX Device"=w344:T4)  [unwired: 9 in, 1 out]
          n232 = call <vilib>:"WPI_EncoderReset.vi"("EncoderDevRef"=w347) -> ("EncoderDevRef"=w346:T6)  [unwired: 9 in, 1 out]
          n233 = call <vilib>:"WPI_EncoderReset.vi"("EncoderDevRef"=w349) -> ("EncoderDevRef"=w348:T6)  [unwired: 9 in, 1 out]
          n234 = while {
            tunnel: w348 -> [_]
            tunnel: w346 -> [_]
            tunnel: w344 -> [w363]
            stop <- w356 stop-if-true
            n235 = call "Z900_navX_Get_YPRHfH.vi"("navX Device"=w363) -> ("YRPHfH"=w362:T10)  [unwired: 7 in, 3 out]
            n236 = call-poly <vilib>:"NT Read Value.vi"("Name"="Position") -> ("Numeric"=w353:dbl)  [unwired: 9 in, 1 out]
            n237 = case shown="Default" w353 {
              tunnel: [0.0 35.0 20.0 0.0 -20.0 -45.0] -> w354
              frame Default {
              }
              frame 1 {
              }
              frame 2 {
              }
              frame 3 {
              }
              frame 4 {
              }
              frame 5 {
              }
            }
            n238 = Unbundle By Name(w362) -> ("Yaw"=w360:dbl)  [unwired: 1 out]
            n239 = local read "Single Turn Gains"() -> (w359:T1)
            n240 = call-poly <vilib>:"PID.vi"("output range"=cluster{"output high":dbl, "output low":dbl} {"output high"=0.8, "output low"=-0.8}, "PID gains"=w359, "process variable"=w360, "setpoint"=w354) -> ("output"=w358:dbl)  [unwired: 6 in, 1 out]
            n241 = local write "Left Motor Speed"(w358) -> ()
            n242 = Multiply(x=-1.0, y=w358) -> (x*y=w357:dbl)
            n243 = local write "Right Motor Speed"(w357) -> ()
            n244 = call <vilib>:"WPI_RobotDriveRefNum Registry Get.vi"("refnum name"="Left and Right Motors") -> ("RobotDriveDevRef"=w366:T11)  [unwired: 9 in, 1 out]
            n245 = call <vilib>:"WPI_RobotDriveTankDrive.vi"("Right axis value"=w358, "Left axis value"=w357, "RobotDriveDevRef"=w366) -> ()  [unwired: 6 in, 3 out]
            n246 = call "Elapsed Time"() -> ("Time has Elapsed"=w356:bool)  [unwired: 12 in, 7 out]
            n247 = Wait (ms)(milliseconds to wait=u32 50) -> ()  [unwired: 1 out]
          }
        }
        frame #2 {
          n248 = while {
            stop <- w384 stop-if-true
            n249 = local read "Aiming Gains"() -> (w374:T1)
            n250 = global read "Robot Global Data.vi" "T1 X"() -> (w382:dbl)
            n251 = Absolute Value(x=w382) -> (abs(x)=w387:dbl)
            n252 = Less?(x=w387, y=0.05) -> (x < y?=w385:bool)
            n253 = call-poly <vilib>:"PID.vi"("output range"=cluster{"output high":dbl, "output low":dbl} {"output high"=0.7, "output low"=-0.7}, "PID gains"=w374, "process variable"=w382, "setpoint"=0.0) -> ("output"=w376:dbl)  [unwired: 6 in, 1 out]
            n254 = case shown="False" w385 {
              tunnel: [FALSE FALSE] -> w384
              frame False {
              }
              frame True {
              }
            }
            n255 = Multiply(x=w376, y=-1.0) -> (x*y=w375:dbl)
            n256 = call <vilib>:"WPI_RobotDriveRefNum Registry Get.vi"("refnum name"="Left and Right Motors") -> ("RobotDriveDevRef"=w378:T11)  [unwired: 9 in, 1 out]
            n257 = call <vilib>:"WPI_RobotDriveTankDrive.vi"("Right axis value"=w375, "Left axis value"=w376, "RobotDriveDevRef"=w378) -> ()  [unwired: 6 in, 3 out]
            n258 = Wait (ms)(milliseconds to wait=u32 50) -> ()  [unwired: 1 out]
          }
        }
      }
    }
    frame "Dashboard Auton" {
      n259 = flat-sequence {
        frame #0 {
          n260 = while {
            stop <- w400 stop-if-true
            n261 = global read "Robot Global Data.vi" "T1 X"() -> (w398:dbl)
            n262 = Absolute Value(x=w398) -> (abs(x)=w403:dbl)
            n263 = Less?(x=w403, y=0.05) -> (x < y?=w401:bool)
            n264 = call-poly <vilib>:"PID.vi"("output range"=cluster{"output high":dbl, "output low":dbl} {"output high"=0.7, "output low"=-0.7}, "PID gains"="Aiming Gains", "process variable"=w398, "setpoint"=0.0) -> ("output"=w391:dbl)  [unwired: 6 in, 1 out]
            n265 = case shown="False" w401 {
              tunnel: [FALSE FALSE] -> w400
              frame False {
              }
              frame True {
              }
            }
            n266 = Multiply(x=w391, y=-1.0) -> (x*y=w390:dbl)
            n267 = call <vilib>:"WPI_RobotDriveRefNum Registry Get.vi"("refnum name"="Left and Right Motors") -> ("RobotDriveDevRef"=w393:T11)  [unwired: 9 in, 1 out]
            n268 = call <vilib>:"WPI_RobotDriveTankDrive.vi"("Right axis value"=w390, "Left axis value"=w391, "RobotDriveDevRef"=w393) -> ()  [unwired: 6 in, 3 out]
            n269 = Wait (ms)(milliseconds to wait=u32 50) -> ()  [unwired: 1 out]
          }
        }
      }
    }
  }
